vi "State Machine - Dequeue State.vi"(6 "Timeout":i32, 8 "error in (no error)":errorcluster, 11 "Queue In":refnum<queue>) -> (0 "error out":errorcluster, 1 "Data":variant, 2 "State":string, 3 "Queue Out":refnum<queue>, 5 "timed out?":bool)   [LabVIEW 2015, in "State Machine.lvlib"]
uses:
  State Machine.lvlib
  Controls/Message.ctl
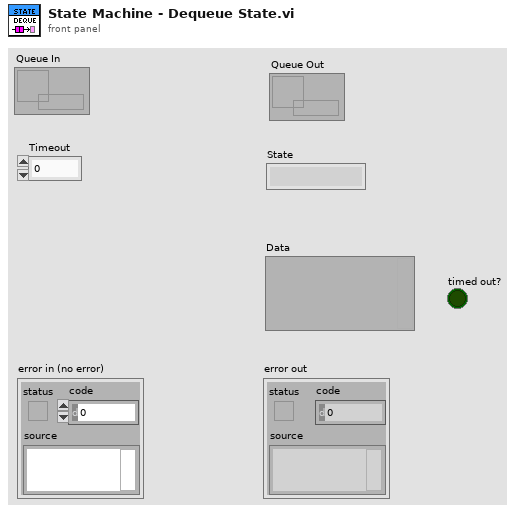
[diagram p1: front panel]
types:
  T1 = typedef "State Machine.lvlib/Message.ctl" = cluster{"State":string, "Data":variant}
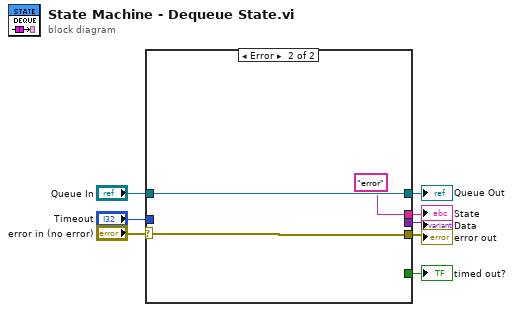
[diagram p0: block diagram]
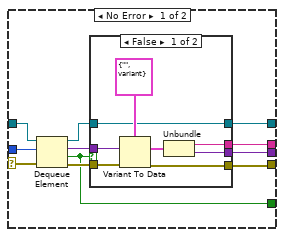
[diagram p2: hidden frame]
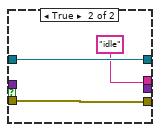
[diagram p3: hidden frame]
diagram:
  n1 = case shown="Error" "error in (no error)" {
    selector: "error in (no error)" -> [w19 w33]
    tunnel: [w12 w33] -> w8
    tunnel: "Queue In" -> [w18 w32]
    tunnel: "Timeout" -> [w17 _]
    tunnel: [w14 "error" ("State")] -> w3
    tunnel: [w13 _] -> w2
    tunnel: [w10 w32] -> w4
    tunnel: [w9 _] -> w1
    frame No Error {
      n2 = Dequeue Element(queue=w18, timeout in ms (-1)=w17, error in (no error)=w19) -> (queue out=w11:refnum<queue>, element=w15:variant, timed out?=w9:bool, error out=w16:errorcluster)
      n3 = case shown="False" w9 {
        tunnel: w16 -> [w27 w28]
        tunnel: w15 -> [w26 _]
        tunnel: [w23 "idle" ("State")] -> w14
        tunnel: [w22 _] -> w13
        tunnel: [w21 w28] -> w12
        tunnel: w11 -> [w20 w30]
        tunnel: [w20 w30] -> w10
        frame False {
          n4 = Variant To Data(error in=w27, type=T1 {"State"="", "Data"=variant} ("Message"), Variant=w26) -> (data=w24:T1, error out=w21:errorcluster)
          n5 = Unbundle(w24) -> ("State"=w23:string, "Data"=w22:variant)
        }
        frame True {
        }
      }
    }
    frame Error {
    }
  }
  "error out" <- w8
  "State" <- w3
  "Data" <- w2
  "Queue Out" <- w4
  "timed out?" <- w1
